vi "Scan_set_delay_list.vi"(0 "Item Names":string[][](array[string]), 1 "Pump":dbl, 3 "Probe":dbl) -> (2 "Delay_full_dir":string[](array[string]), 4 "Delay_dir_list":string[](array[string]), 5 "to_name":string, 6 "Number delays":i32, 7 "Delay_list":dbl[][](array[numeric]), 8 "Delays?":bool, 9 "First Point":dbl)   [LabVIEW 2019]
panel:
  out "No Delays":bool
  out "Final Delay":dbl
  out "size(s)":i32[](array[numeric])
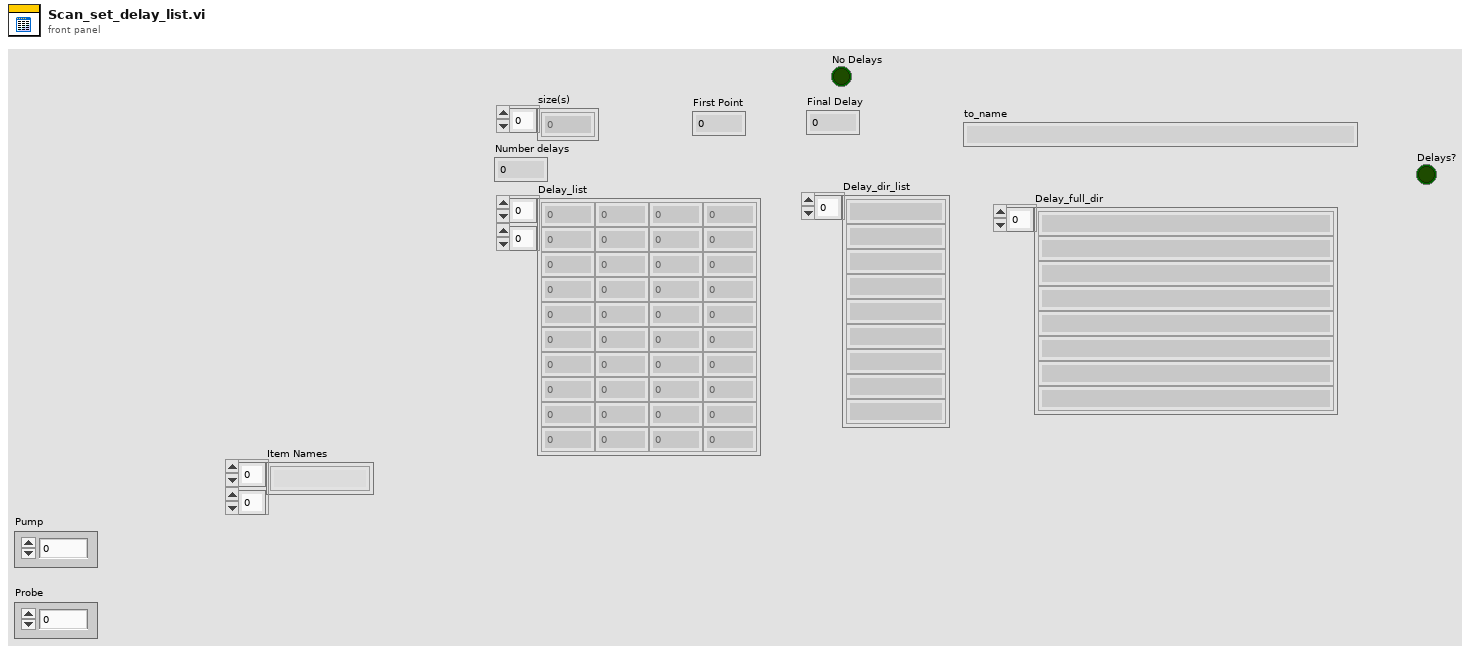
[diagram p1: front panel]
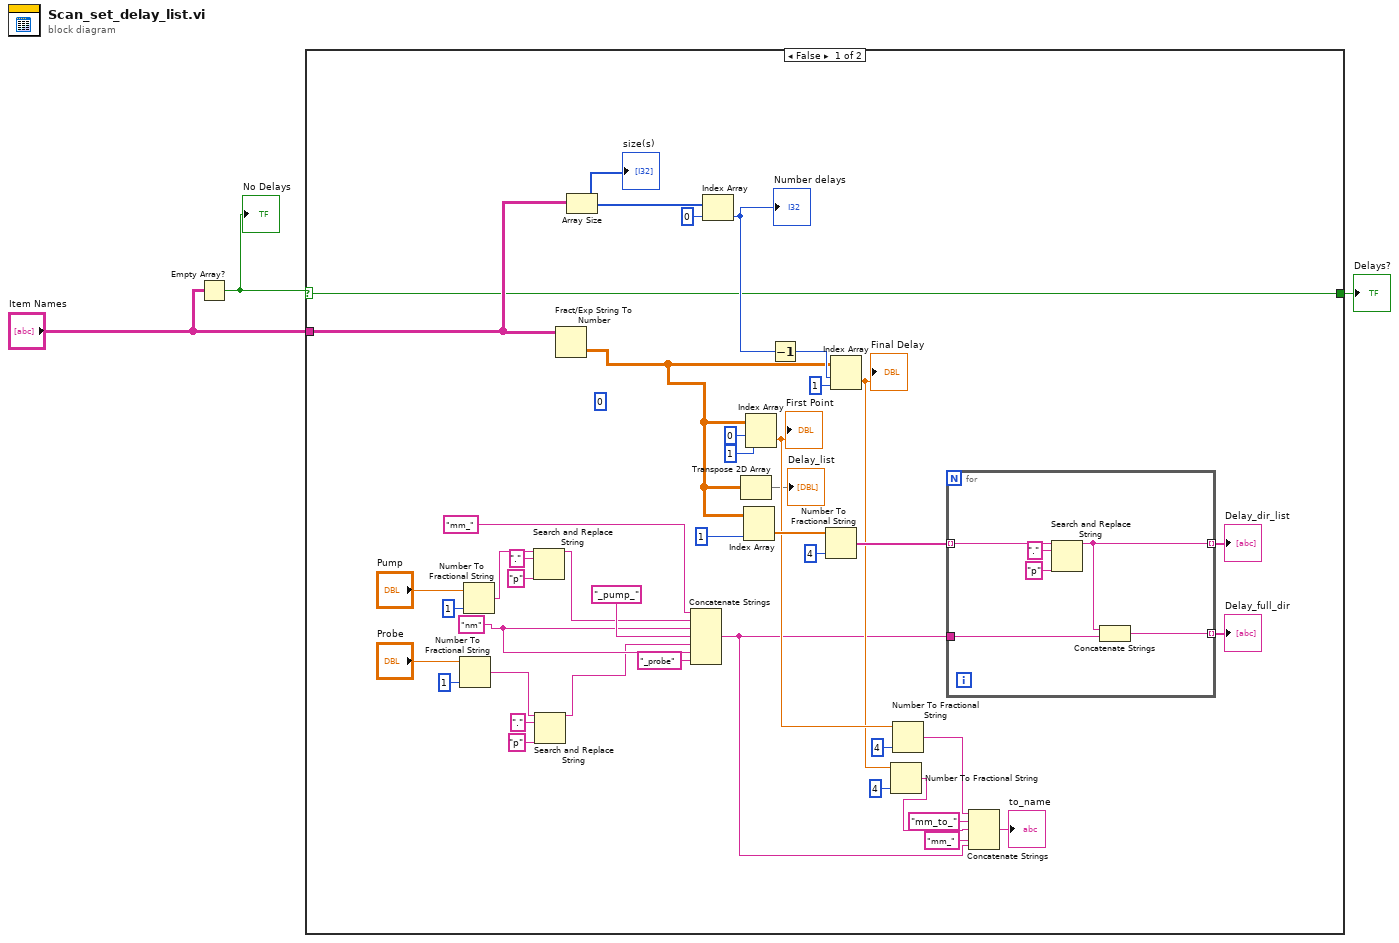
[diagram p0: block diagram]
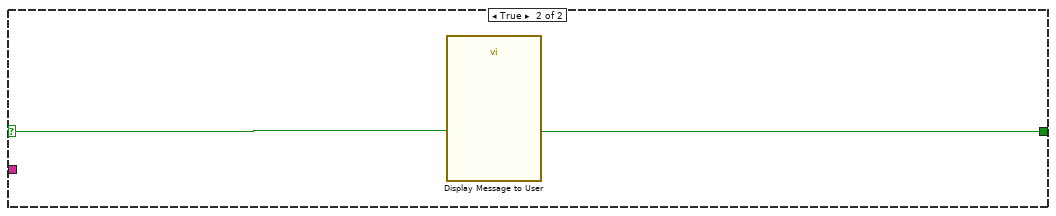
[diagram p2: hidden frame]
diagram:
  n1 = Empty Array?(array="Item Names") -> (empty?=w3:bool)
  "No Delays" <- w3
  n2 = case shown="False" w3 {
    selector: w3 -> [w6 w54]
    tunnel: "Item Names" -> [w7 _]
    tunnel: [w6 w53] -> w2
    frame False {
      w32 = "nm" ("string")
      (unwired) 0 ("index (row)")
      n3 = Number To Fractional String(number="Probe", precision (6)=i16 1) -> (F-format string=w23:string)  [unwired: 2 in]
      n4 = Number To Fractional String(number="Pump", precision (6)=i16 1) -> (F-format string=w27:string)  [unwired: 2 in]
      n5 = Search and Replace String(input string=w27, search string=".", replace string="p" ("replace string (\"\")")) -> (result string=w26:string)  [unwired: 5 in, 3 out]
      n6 = Search and Replace String(input string=w23, search string=".", replace string="p" ("replace string (\"\")")) -> (result string=w22:string)  [unwired: 5 in, 3 out]
      n7 = Fract/Exp String To Number(string=w7) -> (number=w5:dbl[][])  [unwired: 3 in, 1 out]
      n8 = Array Size(array=w7) -> (size(s)=w46:i32[])
      "size(s)" <- w46
      n9 = Concatenate Strings("mm_", w26, w32, "_pump_" ("string"), w22, w32, "_probe" ("string")) -> (w9:string)
      n10 = Index Array(array=w46, index=0) -> (element=w19:i32)
      "Number delays" <- w19
      n11 = Transpose 2D Array(2D array=w5) -> (transposed array=→"Delay_list":dbl[][])
      n12 = Index Array(array=w5, index (col)=1 ("index (row)")) -> (element=w41:dbl[])  [unwired: 1 in]
      n13 = Index Array(array=w5, index (row)=0, index (col)=1 ("disabled index (col)")) -> (element=w15:dbl)
      "First Point" <- w15
      n14 = Decrement(x=w19) -> (x-1=w18:i32)
      n15 = Number To Fractional String(number=w41, precision (6)=i16 4) -> (F-format string=w40:string[])  [unwired: 2 in]
      n16 = Index Array(array=w5, index (row)=w18, index (col)=1 ("disabled index (col)")) -> (element=w14:dbl)
      "Final Delay" <- w14
      n17 = Number To Fractional String(number=w14, precision (6)=i16 4) -> (F-format string=w11:string)  [unwired: 2 in]
      n18 = Number To Fractional String(number=w15, precision (6)=i16 4) -> (F-format string=w13:string)  [unwired: 2 in]
      n19 = for {
        tunnel: w40 -> [w52] mode=indexing
        tunnel: [w48] -> w39 mode=indexing
        tunnel: w9 -> [w49]
        tunnel: [w47] -> w30 mode=indexing
        n20 = Search and Replace String(input string=w52, search string=".", replace string="p" ("replace string (\"\")")) -> (result string=w48:string)  [unwired: 5 in, 3 out]
        n21 = Concatenate Strings(w48, w49) -> (w47:string)
      }
      "Delay_dir_list" <- w39
      "Delay_full_dir" <- w30
      n22 = Concatenate Strings(w13, "mm_to_" ("string"), w11, "mm_" ("string"), w9) -> (→"to_name":string)
    }
    frame True {
      n23 = call "Display Message to User"("Enable"=w54) -> ("OK"=w53:bool)  [unwired: 9 in, 1 out]
    }
  }
  "Delays?" <- w2
